vi "Remove File Extensions.vi"(10 "String":string) -> (2 "String out":string)   [LabVIEW 2017, in "Cobertura.lvlib"]
uses:
  Cobertura.lvlib
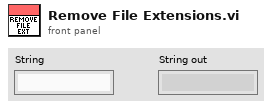
[diagram p1: front panel]
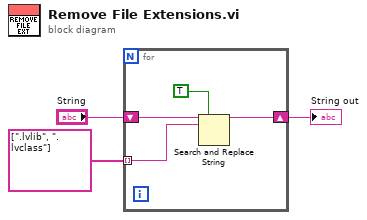
[diagram p0: block diagram]
diagram:
  n1 = for {
    shift-right: [w5] -> w2
    shift-left: "String" -> [w7]
    tunnel: string[] [".lvlib", ".lvclass"] -> [w4] mode=indexing
    n2 = Search and Replace String(replace all?=TRUE ("replace all? (F)"), input string=w7, search string=w4) -> (result string=w5:string)  [unwired: 5 in, 3 out]
  }
  "String out" <- w2
